vi "current_folder.vi"(10 "extension":string, 11 "filename":string) -> (3 "Path":path)   [LabVIEW 2013]
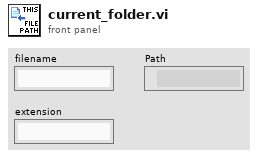
[diagram p1: front panel]
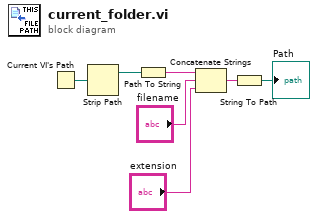
[diagram p0: block diagram]
diagram:
  n1 = Current VI's Path() -> (path=w3:path)
  n2 = Strip Path(path=w3) -> (stripped path=w2:path)  [unwired: 1 out]
  n3 = Path To String(path=w2) -> (string=w1:string)
  n4 = Concatenate Strings(w1, "filename", "extension") -> (w6:string)
  n5 = String To Path(string=w6) -> (path=→"Path":path)
